vi "LVMark_TestString.vi"() -> ()   [LabVIEW 2009]
uses:
  LVMark_optype.ctl
  LVMark_opcluster.ctl
panel:
  in  "Input string":string="Supported items:\n**text** = bold text\n__text__ = bold text\n*text* = italic text\n_text_ = italic text\n[#5D8AA8]text[#5D8AA8] = Air Force blue text\n[#CD9575]text[#CD9575] = Antique brass text\n[#FF033E]text[#FF033E] = American rose text\n[verysmall]text[verysmall] = very small text\n[small]text[small] = small text\n[large]text[large] = large text\n[verylarge]text[verylarge] = very large text\n[sys]text[sys] = system font\n[app]text[app] = application font\n[dlg]text[dlg] = dialog font\n[arial]text[arial] = arial font\n[times new roman]text[times new roman] = times new roman font\n[s]text[s] = strikethrough text\n[strike]text[strike] = strikethrough text\n[u]text[u] = underline text\n[under]text[under] = underline text\n\n*Lorem ipsum dolor sit amet*, **consectetur adipiscing elit**. Cras vehicula velit quis purus aliquam lacinia. Curabitur convallis mi at lectus commodo scelerisque. Sed ultrices odio velit. *[#CD9575]In sodales, leo non adipiscing aliquam[#CD9575]*, velit turpis auctor velit, eu pulvinar massa turpis a urna. Aliquam viverra, erat ac sodales aliquet, tortor ipsum mattis elit, non pharetra enim turpis pretium leo. [small]Duis risus augue, mollis ut congue vel, mattis in velit. Phasellus interdum eros id nisl euismod sed cursus dui pellentesque.[small] [large]Aliquam[large] placerat, odio vitae elementum facilisis, diam justo porta dolor, sit amet tincidunt neque lorem quis ante. Aliquam porta, orci ac [arial]mattis suscipit, odio enim lacinia libero, quis sagittis lacus risus[arial] eu metus. Morbi vel massa mauris, vitae fringilla sem. Praesent eget est purus. Etiam viverra [#FF033E]tempor libero at __convallis. _In hac_ habitas__se platea dictumst. Quisque metus justo, varius vitae volutpat ac, euismod eget metus. Mauris metus ligula, ornare eu[#FF033E] interdum id, lobortis vel elit. Proin vehicula quam eu erat sodales quis tempus orci ultrices. Maecenas elementum odio in quam facilisis in bibendum [verysmall]mi[verysmall] [verylarge]elementum[verylarge]."
  out "Output String":string="Test\nthis is a test\nonly a test\nof the bold\nand the italic\nand the font\nand the color"
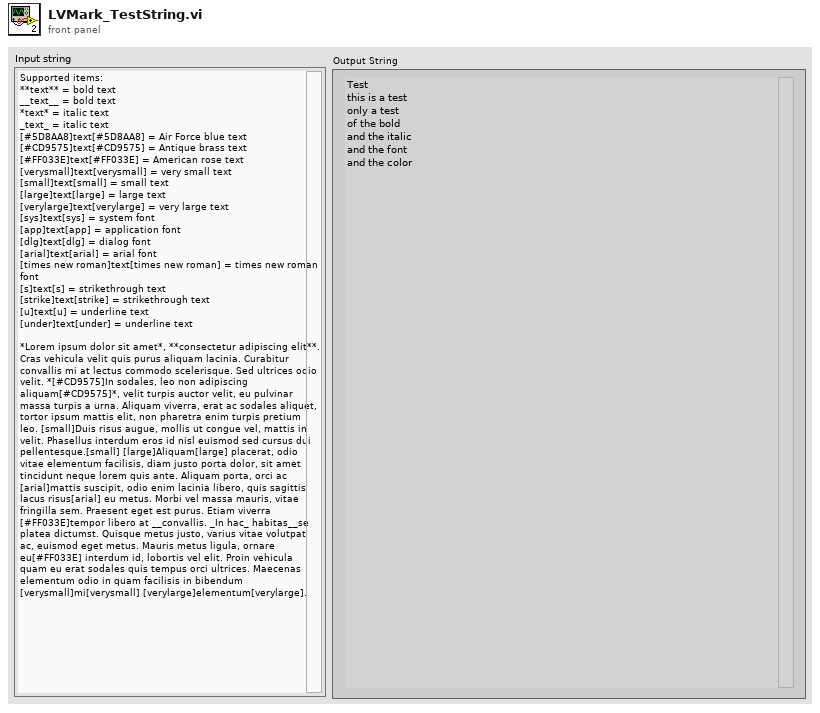
[diagram p1: front panel]
types:
  T1 = typedef "LVMark_optype.ctl" = enum16{"bold", "italic", "underline", "color", "font", "fontsize", "strikethrough"}
  T2 = typedef "LVMark_opcluster.ctl" = cluster{"optype":T1, "params":string, "selstart":i32, "selend":i32}
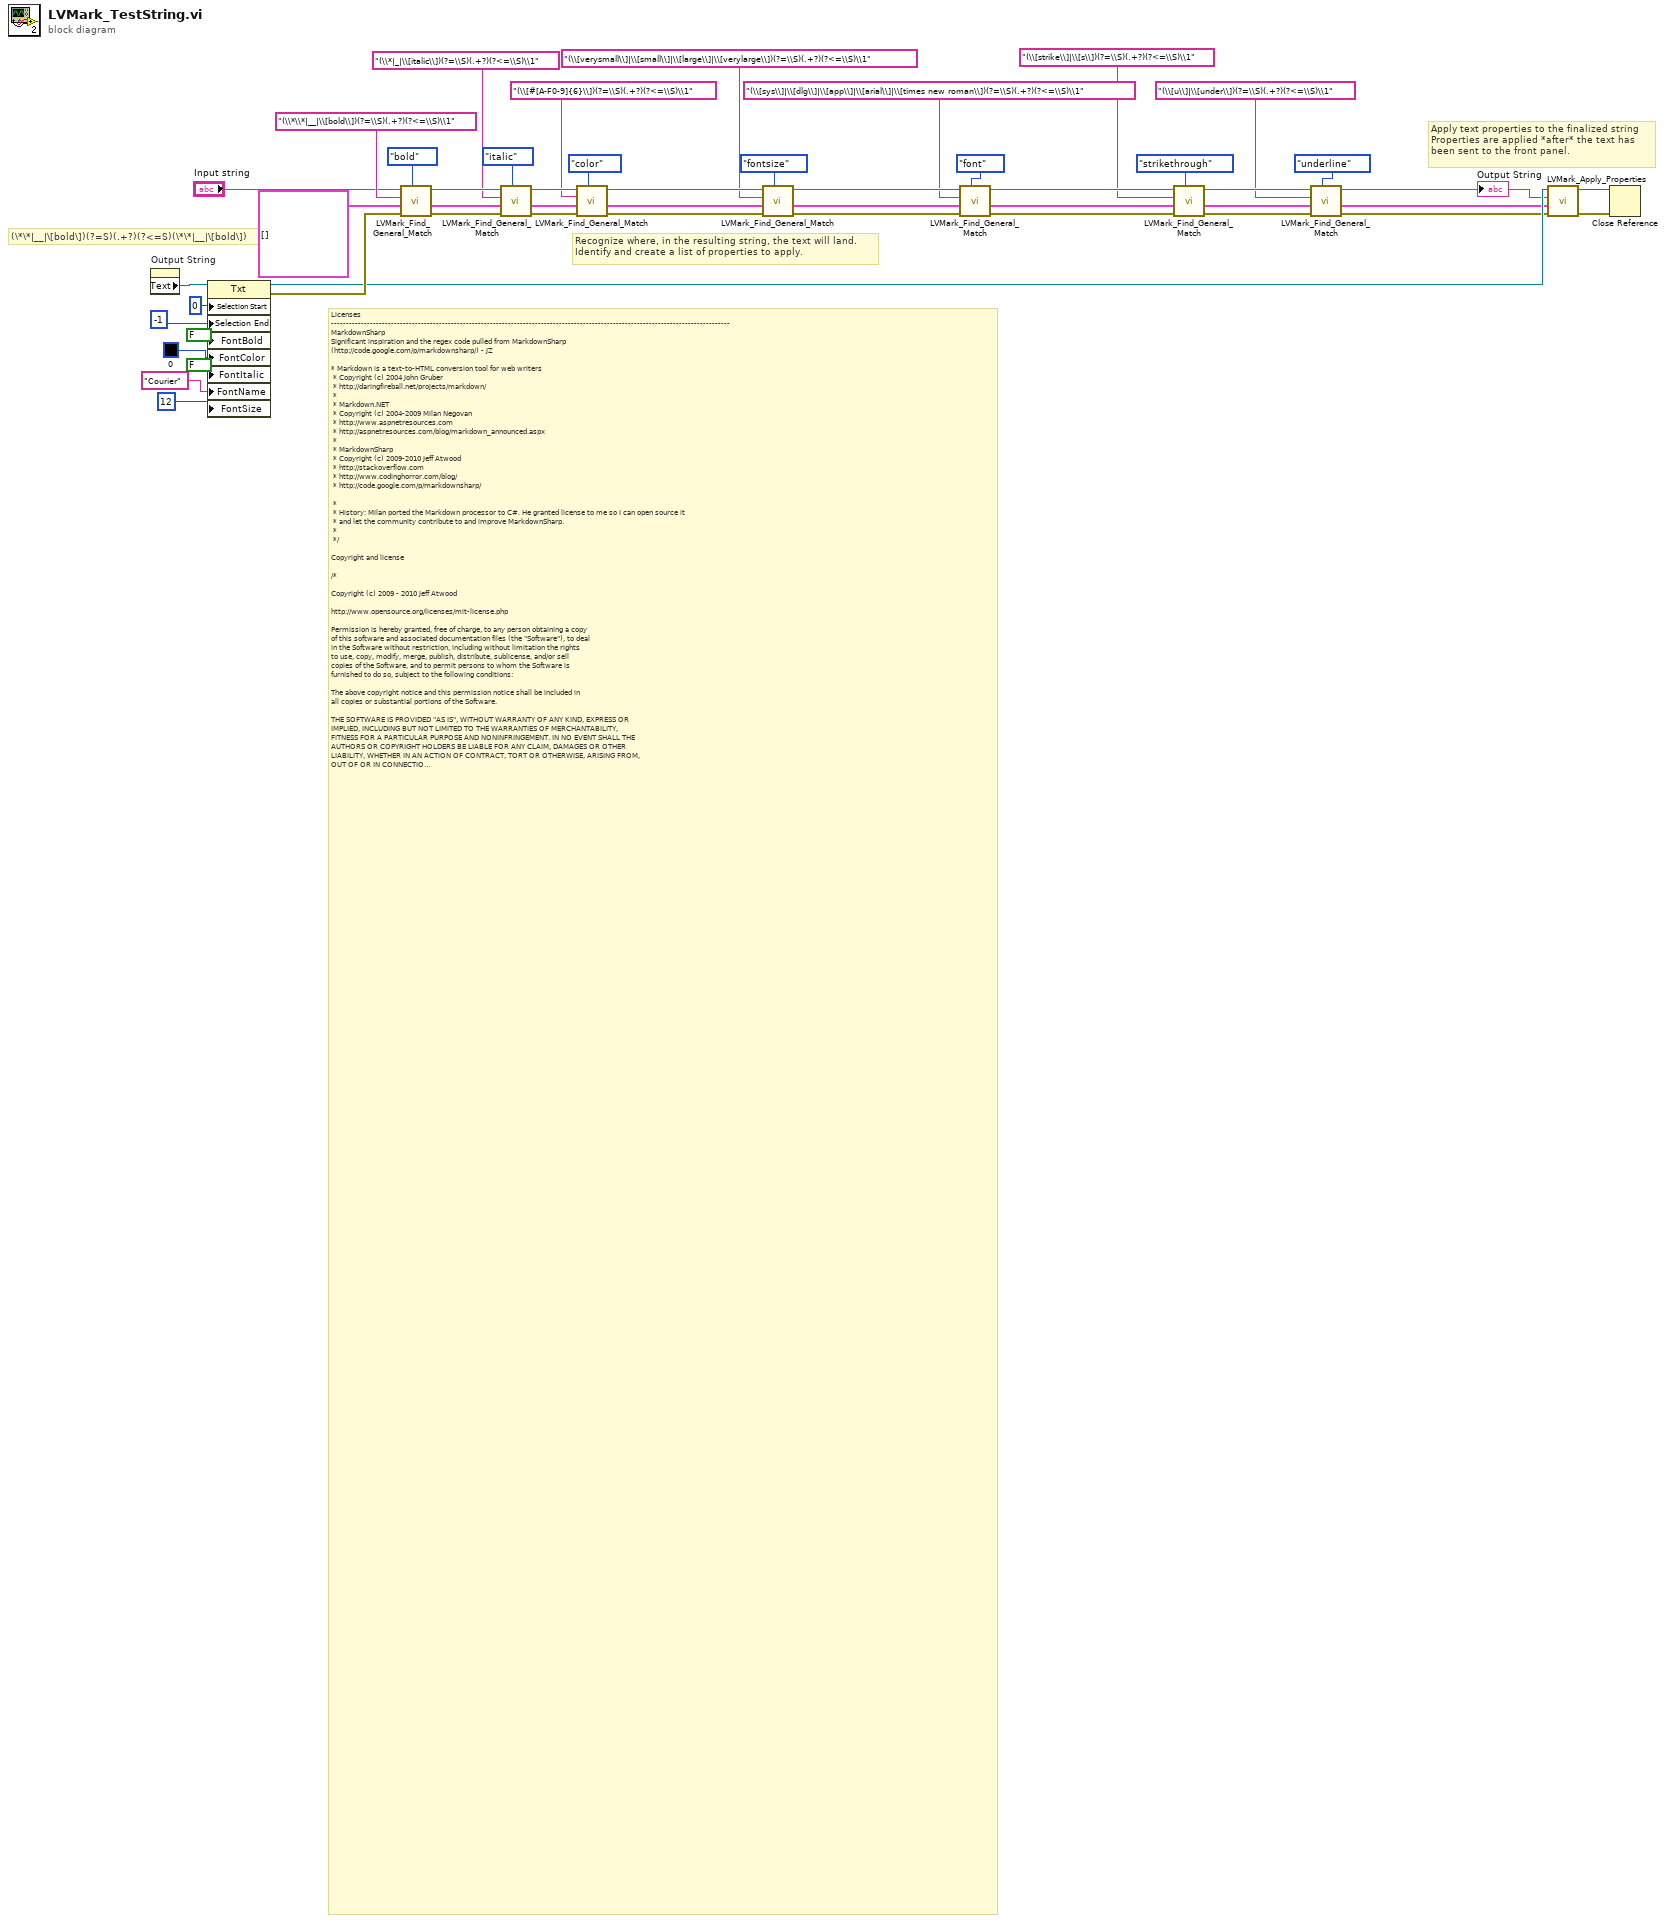
[diagram p0: block diagram]
diagram:
  # "Apply text properties to the finalized string\nProperties are applied *after* the text has\nbeen sent to the front panel."
  # "Recognize where, in the resulting string, the text will land.\nIdentify and create a list of properties to apply."
  # "Licenses\n-------------------------------------------------------------------------------------------------------------------------------------\nMarkdownSharp\nSignificant inspiration and the regex code pulled from MarkdownSharp\n(http://code.google.com/p/markdownsharp/) - JZ\n\n* Markdown is a text-to-HTML conversion tool for web writers\n * Copyright (c) 2004 John Gruber\n * http://daringfireball.net/projects/markdown/\n * \n * Markdown.NET\n * Copyright (c) 2004-2009 Milan Negovan\n * http://www.aspnetresources.com\n * http://aspnetresources.com/blog/markdown_announced.aspx\n * \n * MarkdownSharp\n * Copyright (c) 2009-2010 Jeff Atwood\n * http://stackoverflow.com\n * http://www.codinghorror.com/blog/\n * http://code.google.com/p/markdownsharp/\n\n * \n * History: Milan ported the Markdown processor to C#. He granted license to me so I can open source it\n * and let the community contribute to and improve MarkdownSharp.\n * \n */\n\nCopyright and license\n\n/*\n\nCopyright (c) 2009 - 2010 Jeff Atwood\n\nhttp://www.opensource.org/licenses/mit-license.php\n  \nPermission is hereby granted, free of charge, to any person obtaining a copy\nof this software and associated documentation files (the \"Software\"), to deal\nin the Software without restriction, including without limitation the rights\nto use, copy, modify, merge, publish, distribute, sublicense, and/or sell\ncopies of the Software, and to permit persons to whom the Software is\nfurnished to do so, subject to the following conditions:\n\nThe above copyright notice and this permission notice shall be included in\nall copies or substantial portions of the Software.\n\nTHE SOFTWARE IS PROVIDED \"AS IS\", WITHOUT WARRANTY OF ANY KIND, EXPRESS OR\nIMPLIED, INCLUDING BUT NOT LIMITED TO THE WARRANTIES OF MERCHANTABILITY,\nFITNESS FOR A PARTICULAR PURPOSE AND NONINFRINGEMENT. IN NO EVENT SHALL THE\nAUTHORS OR COPYRIGHT HOLDERS BE LIABLE FOR ANY CLAIM, DAMAGES OR OTHER\nLIABILITY, WHETHER IN AN ACTION OF CONTRACT, TORT OR OTHERWISE, ARISING FROM,\nOUT OF OR IN CONNECTION WITH THE SOFTWARE OR THE USE OR OTHER DEALINGS IN\nTHE SOFTWARE.\n\nCopyright (c) 2003-2004 John Gruber\n<http://daringfireball.net/>   \nAll rights reserved.\n\nRedistribution and use in source and binary forms, with or without\nmodification, are permitted provided that the following conditions are\nmet:\n\n* Redistributions of source code must retain the above copyright notice,\n  this list of conditions and the following disclaimer.\n\n* Redistributions in binary form must reproduce the above copyright\n  notice, this list of conditions and the following disclaimer in the\n  documentation and/or other materials provided with the distribution.\n\n* Neither the name \"Markdown\" nor the names of its contributors may\n  be used to endorse or promote products derived from this software\n  without specific prior written permission.\n\nThis software is provided by the copyright holders and contributors \"as\nis\" and any express or implied warranties, including, but not limited\nto, the implied warranties of merchantability and fitness for a\nparticular purpose are disclaimed. In no event shall the copyright owner\nor contributors be liable for any direct, indirect, incidental, special,\nexemplary, or consequential damages (including, but not limited to,\nprocurement of substitute goods or services; loss of use, data, or\nprofits; or business interruption) however caused and on any theory of\nliability, whether in contract, strict liability, or tort (including\nnegligence or otherwise) arising in any way out of the use of this\nsoftware, even if advised of the possibility of such damage.\n*/\n-------------------------------------------------------------------------------------------------------------------------------------\nLVMark\n\nThe (non-NI) LabVIEW portions of the code are:\n\nCopyright (c) 2011 Joe Zoller\njoe@underflowsoftware.com\n\nhttp://www.opensource.org/licenses/mit-license.php).\nPermission is hereby granted, free of charge, to any person obtaining a copy of this software and associated\ndocumentation files (the \"Software\"), to deal in the Software without restriction, including without limitation the\nrights to use, copy, modify, merge, publish, distribute, sublicense, and/or sell copies of the Software, and to\npermit persons to whom the Software is furnished to do so, subject to the following conditions:\n\nThe above copyright notice and this permission notice shall be included in all copies or substantial portions of\nthe Software.\n\nTHE SOFTWARE IS PROVIDED \"AS IS\", WITHOUT WARRANTY OF ANY KIND, EXPRESS OR IMPLIED,\nINCLUDING BUT NOT LIMITED TO THE WARRANTIES OF MERCHANTABILITY, FITNESS FOR A PARTICULAR\nPURPOSE AND NONINFRINGEMENT. IN NO EVENT SHALL THE AUTHORS OR COPYRIGHT HOLDERS BE LIABLE\nFOR ANY CLAIM, DAMAGES OR OTHER LIABILITY, WHETHER IN AN ACTION OF CONTRACT, TORT OR\nOTHERWISE, ARISING FROM, OUT OF OR IN CONNECTION WITH THE SOFTWARE OR THE USE OR OTHER\nDEALINGS IN THE SOFTWARE."
  # "(\\*\\*|__|\\[bold\\])(?=S)(.+?)(?<=S)(\\*\\*|__|\\[bold\\])"
  n1 = property on="Output String" class="Str"() -> ("Text"=w46:refnum<vi>)  [unwired: 2 in, 2 out]
  n2 = property class="Txt"(reference=w46, "Selection Start"=u32 0 ("Selection:Start"), "Selection End"=-1 ("Selection:Start"), "FontBold"=FALSE ("Font:Bold"), "FontColor"=u32 0, "FontItalic"=FALSE ("Font:Italic"), "FontName"="Courier" ("Font:Name"), "FontSize"=u32 12 ("Font:Size")) -> (reference out=w31:refnum<vi>, error out=w39:errorcluster)  [unwired: 1 in]
  n3 = call "LVMark_Find_General_Match.vi"("optype"=LVMark_optype."bold", "error in"=w39, "Operations"=T2[] [], "regular expression"="(\\*\\*|__|\\[bold\\])(?=\\S)(.+?)(?<=\\S)\\1", "ML string"="Input string") -> ("error out"=w35:errorcluster, "Operations out"=w32:T2[], "ML string out"=w38:string)  [unwired: 4 in]
  n4 = call "LVMark_Find_General_Match.vi"("optype"=LVMark_optype."italic", "error in"=w35, "Operations"=w32, "regular expression"="(\\*|_|\\[italic\\])(?=\\S)(.+?)(?<=\\S)\\1", "ML string"=w38) -> ("error out"=w30:errorcluster, "Operations out"=w28:T2[], "ML string out"=w29:string)  [unwired: 4 in]
  n5 = call "LVMark_Find_General_Match.vi"("optype"=LVMark_optype."color", "error in"=w30, "Operations"=w28, "regular expression"="(\\[#[A-F0-9]{6}\\])(?=\\S)(.+?)(?<=\\S)\\1", "ML string"=w29) -> ("error out"=w24:errorcluster, "Operations out"=w22:T2[], "ML string out"=w23:string)  [unwired: 4 in]
  n6 = call "LVMark_Find_General_Match.vi"("optype"=LVMark_optype."fontsize", "error in"=w24, "Operations"=w22, "regular expression"="(\\[verysmall\\]|\\[small\\]|\\[large\\]|\\[verylarge\\])(?=\\S)(.+?)(?<=\\S)\\1", "ML string"=w23) -> ("error out"=w19:errorcluster, "Operations out"=w18:T2[], "ML string out"=w17:string)  [unwired: 4 in]
  n7 = call "LVMark_Find_General_Match.vi"("optype"=LVMark_optype."font", "error in"=w19, "Operations"=w18, "regular expression"="(\\[sys\\]|\\[dlg\\]|\\[app\\]|\\[arial\\]|\\[times new roman\\])(?=\\S)(.+?)(?<=\\S)\\1", "ML string"=w17) -> ("error out"=w14:errorcluster, "Operations out"=w13:T2[], "ML string out"=w12:string)  [unwired: 4 in]
  n8 = call "LVMark_Find_General_Match.vi"("optype"=LVMark_optype."strikethrough", "error in"=w14, "Operations"=w13, "regular expression"="(\\[strike\\]|\\[s\\])(?=\\S)(.+?)(?<=\\S)\\1", "ML string"=w12) -> ("error out"=w5:errorcluster, "Operations out"=w6:T2[], "ML string out"=w7:string)  [unwired: 4 in]
  n9 = call "LVMark_Find_General_Match.vi"("optype"=LVMark_optype."underline", "error in"=w5, "Operations"=w6, "regular expression"="(\\[u\\]|\\[under\\])(?=\\S)(.+?)(?<=\\S)\\1", "ML string"=w7) -> ("error out"=w2:errorcluster, "Operations out"=w1:T2[], "ML string out"=w3:string)  [unwired: 4 in]
  "Output String" <- w3
  n10 = call "LVMark_Apply_Properties.vi"("error in"=w2, "Operations"=w1, "ML string"=w3, "Text ref in"=w31) -> ("error out"=w10:errorcluster, "Text ref out"=w9:refnum<vi>)  [unwired: 6 in]
  n11 = Close Reference(reference=w9, error in (no error)=w10) -> ()  [unwired: 1 out]
